vi "Initialize Launch Position.vi"(8 "error in":errorcluster, 11 "Flex Dialog in":refnum<class "Flex UI Dialog.lvclass">) -> (0 "error out":errorcluster, 3 "Flex Dialog out":refnum<class "Flex UI Dialog.lvclass">)   [LabVIEW 2016, in "Flex UI Dialog.lvclass"]
uses:
  Flex UI Dialog.lvclass
  C:/VI Packages/Flex UI/Flex UI (Parent)/Flex UI.lvclass
  Flex UI Dialog.lvclass/Flex UI Dialog.ctl
  Flex UI (Parent)/Flex UI.lvclass/Flex UI.ctl
  Flex UI (Parent)/Flex UI.lvclass
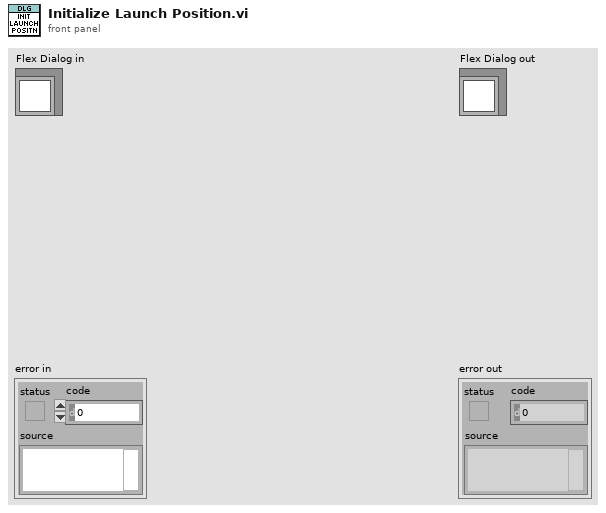
[diagram p1: front panel]
types:
  T1 = typedef "Flex UI Dialog.lvclass/Enum - Launch Position.ctl" = enum16{"Default (Last Opened)", "Centered", "Centered on Caller", "Maximized", "Hidden"}
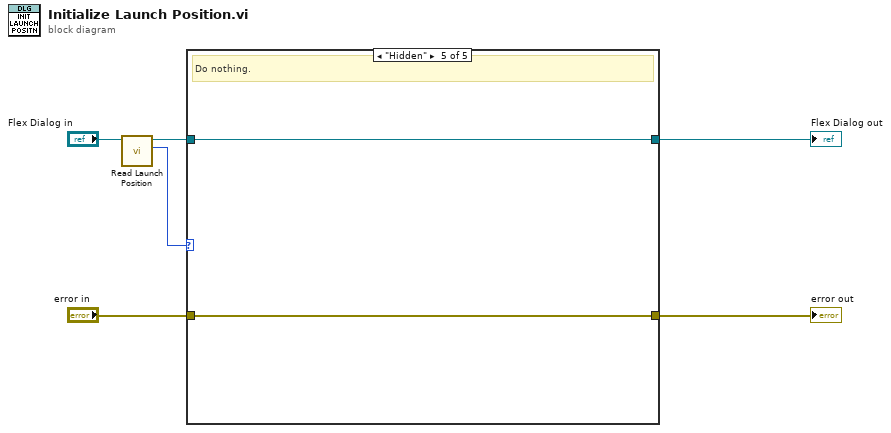
[diagram p0: block diagram]
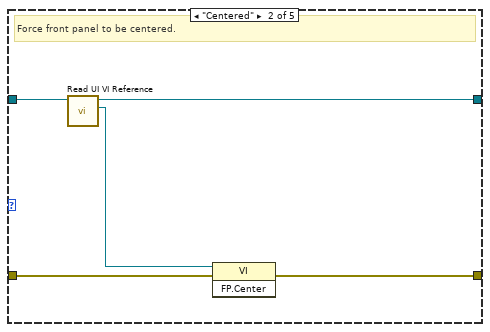
[diagram p3: hidden frame]
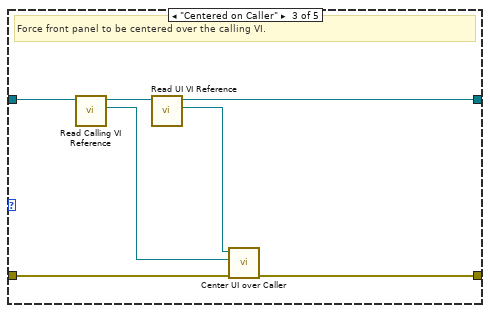
[diagram p4: hidden frame]
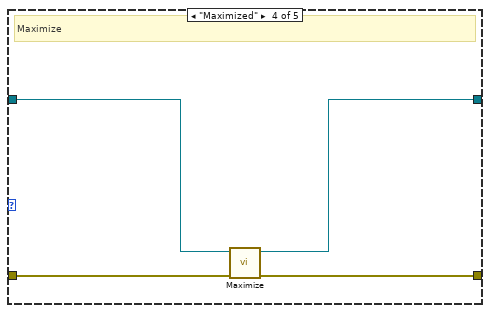
[diagram p5: hidden frame]
diagram:
  n1 = call "Read Launch Position.vi"("Flex Dialog in"="Flex Dialog in") -> ("Launch Position"=w5:T1, "Flex Dialog out"=w3:refnum<class "Flex UI Dialog.lvclass">)  [unwired: 9 in]
  n2 = case shown="\"Hidden\"" w5 {
    tunnel: [w7 w11 w18 w21 w25] -> w4
    tunnel: w3 -> [w7 w13 w20 w22 w25]
    tunnel: [w8 w10 w17 w23 w26] -> w2
    tunnel: "error in" -> [w8 w12 w19 w24 w26]
    frame "Default (Last Opened)", Default {
      # "By defualt, allow dialog to open where it was last saved."
    }
    frame "Centered" {
      # "Force front panel to be centered."
      n3 = call "Read UI VI Reference.vi"("Flex UI in"=w13) -> ("UI VI Reference"=w9:refnum<vi>, "Flex UI out"=w11:refnum<class "Flex UI Dialog.lvclass">)  [unwired: 9 in]
      n4 = invoke class="VI" method="FP.Center"(reference=w9, error in=w12) -> (error out=w10:errorcluster)  [unwired: 1 in, 2 out]
    }
    frame "Centered on Caller" {
      # "Force front panel to be centered over the calling VI."
      n5 = call "Read Calling VI Reference.vi"("Flex Dialog in"=w20) -> ("Calling VI Reference"=w14:refnum<vi>, "Flex Dialog out"=w15:refnum<class "Flex UI Dialog.lvclass">)  [unwired: 9 in]
      n6 = call "Read UI VI Reference.vi"("Flex UI in"=w15) -> ("UI VI Reference"=w16:refnum<vi>, "Flex UI out"=w18:refnum<class "Flex UI Dialog.lvclass">)  [unwired: 9 in]
      n7 = call "Center UI over Caller.vi"("error in"=w19, "Calling VI"=w14, "VI to Center"=w16) -> ("error out"=w17:errorcluster)  [unwired: 8 in]
    }
    frame "Maximized" {
      # "Maximize"
      n8 = call-dynamic "Maximize.vi"("error in"=w24, "Flex Dialog in"=w22) -> ("error out"=w23:errorcluster, "Flex Dialog out"=w21:refnum<class "Flex UI Dialog.lvclass">)  [unwired: 8 in]
    }
    frame "Hidden" {
      # "Do nothing."
    }
  }
  "error out" <- w2
  "Flex Dialog out" <- w4
